vi "Default Timeout.vi"() -> (0 "Timeout":i32)   [LabVIEW 2018]
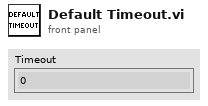
[diagram p1: front panel]
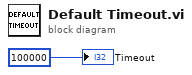
[diagram p0: block diagram]
diagram:
  "Timeout" <- 100000
